vi "Create Licence Key (bidirectional).vi"(8 "error in (no error)":errorcluster, 9 "features (optional)":T1, 10 "application name":string, 11 "machine ID":string) -> (0 "error out":errorcluster, 3 "licence key":string)   [LabVIEW 2013]
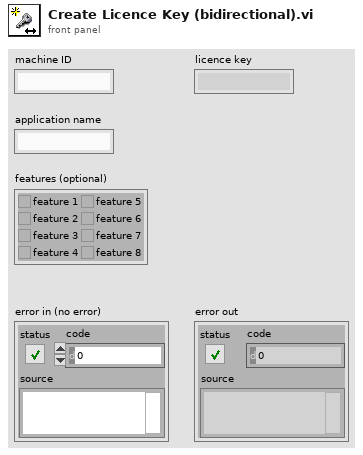
[diagram p1: front panel]
types:
  T1 = cluster{"Feature 1":bool, "Feature 2":bool, "Feature 3":bool, "Feature 4":bool, "Feature 5":bool, "Feature 6":bool, "Feature 7":bool, "Feature 8":bool}
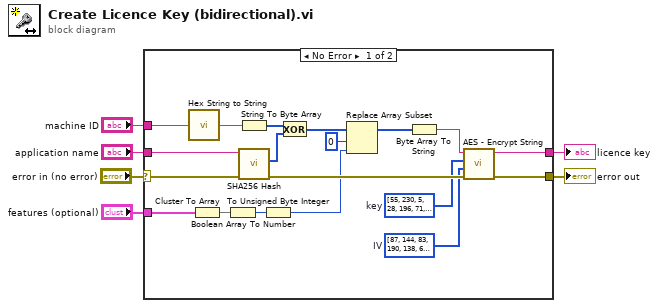
[diagram p0: block diagram]
diagram:
  n1 = case shown="No Error" "error in (no error)" {
    selector: "error in (no error)" -> [w7 w26]
    tunnel: "application name" -> [w25 _]
    tunnel: [w24 w26] -> w5
    tunnel: "features (optional)" -> [w20 _]
    tunnel: [w15 _] -> w3
    tunnel: "machine ID" -> [w8 _]
    frame No Error {
      w13 = u8[] [87, 144, 83, 190, 138, 60, 134, 171, 59, 5, 116, 127, 154, 250, 25, 24]  # IV
      w14 = u8[] [55, 230, 5, 28, 196, 71, 246, 204, 4, 31, 53, 16, 0, 203, 136, 242, 182, 15, 199, 174, 127, 6, 27, 184, 229, 147, 86, 4, 208, 54, 91, 185]  # key
      n2 = call "Hex String to String.vi"("hex string"=w8) -> ("string"=w18:string)
      n3 = Cluster To Array(cluster=w20) -> (array=w22:bool[])
      n4 = Boolean Array To Number(Boolean array=w22) -> (number=w21:u32)
      n5 = String To Byte Array(string=w18) -> (unsigned byte array=w19:u8[])
      n6 = call "SHA256 Hash.vi"("error in (no error)"=w7, "string to hash"=w25) -> ("error out"=w23:errorcluster, "hash bytes"=w11:u8[])  [unwired: 7 in, 1 out]
      n7 = To Unsigned Byte Integer(number=w21) -> (unsigned 8bit integer=w16:u8)
      n8 = Exclusive Or(1:w11, 2:w19) -> (0:w9:u8[])
      n9 = Replace Array Subset(array=w9, new element=w16, index=0) -> (w17:u8[])
      n10 = Byte Array To String(unsigned byte array=w17) -> (string=w10:string)
      n11 = call "AES - Encrypt String.vi"("error in (no error)"=w23, "IV"=w13, "key"=w14, "string to encrypt"=w10) -> ("error out"=w24:errorcluster, "encrypted string"=w15:string)  [unwired: 6 in]
    }
    frame Error {
    }
  }
  "licence key" <- w3
  "error out" <- w5
